vi "Open API Tester.vi"(6 "Run API Tester?":bool, 8 "error in":errorcluster, 10 "Library":refnum<class "Library.lvclass">, 11 "Project":refnum<class "Project.lvclass">) -> (0 "error out":errorcluster)   [LabVIEW 2020, in "Panther Dashboard.lvlib"]
doc: "This VI checks the Main.vi State of the selected DQMH Module"
uses:
  Panther Dashboard.lvlib
  Class/Project/Project.lvclass
  Class/Library/Library.lvclass
  Class/Project/Project.lvclass/Project.ctl
  Class/Library/Library.lvclass/Library.ctl
  Class/Project/Read Main App Inst Ref.vi
  Class/Project/Read Target Name.vi
  Class/Library/Read Library Ref.vi
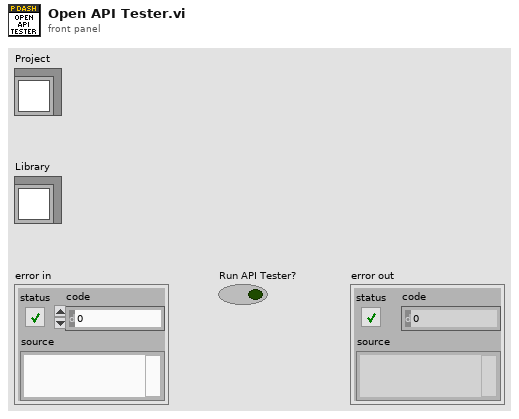
[diagram p1: front panel]
types:
  T1 = enum32{"Bad", "Idle", "Run top level", "Running"}
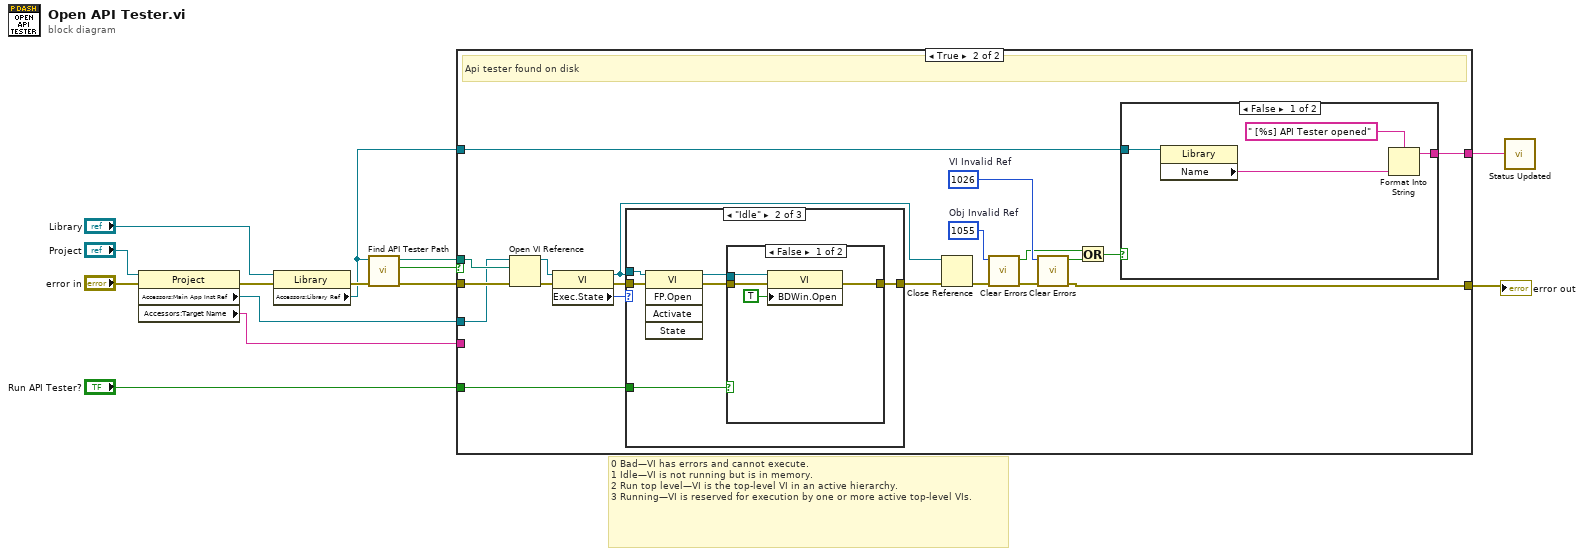
[diagram p0: block diagram]
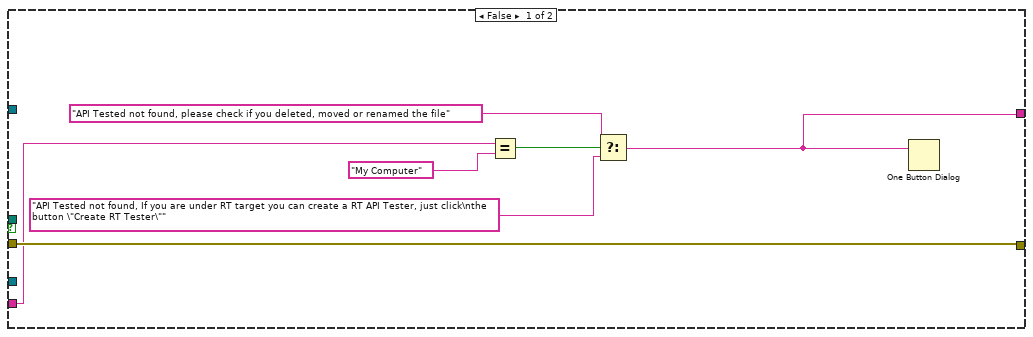
[diagram p2: hidden frame]
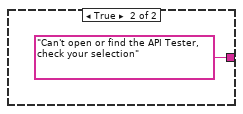
[diagram p3: hidden frame]
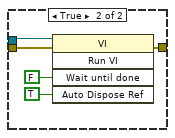
[diagram p5: hidden frame]
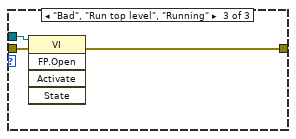
[diagram p6: hidden frame]
diagram:
  # "0\tBad—VI has errors and cannot execute.\n1\tIdle—VI is not running but is in memory.\n2\tRun top level—VI is the top-level VI in an active hierarchy.\n3\tRunning—VI is reserved for execution by one or more active top-level VIs."
  n1 = property class="Project"(reference="Project", error in="error in") -> (error out=w10:errorcluster, "Accessors:Main App Inst Ref"=w3:refnum<vi>, "Accessors:Target Name"=w2:string)  [unwired: 1 out]
  n2 = property class="Library"(reference="Library", error in=w10) -> (error out=w11:errorcluster, "Accessors:Library Ref"=w5:refnum<vi>)  [unwired: 1 out]
  n3 = call "Find API Tester Path.vi"("error in"=w11, "DQMH Library Ref"=w5) -> ("error out"=w13:errorcluster, "Api tester found?"=w8:bool, "API Tester Path"=w9:path)  [unwired: 7 in]
  n4 = case shown="True" w8 {
    tunnel: w13 -> [w21 w40]
    tunnel: w9 -> [_ w34]
    tunnel: w5 -> [_ w25]
    tunnel: w3 -> [_ w24]
    tunnel: [w21 w35] -> w12
    tunnel: [w16 w23] -> w7
    tunnel: w2 -> [w15 _]
    tunnel: "Run API Tester?" -> [_ w22]
    frame False {
      n5 = Equal?(x=w15, y="My Computer") -> (x = y?=w19:bool)
      n6 = Select(t="API Tested not found, please check if you deleted, moved or renamed the file", s=w19, f="API Tested not found, If you are under RT target you can create a RT API Tester, just click\nthe button \"Create RT Tester\"") -> (s? t:f=w16:string)
      n7 = One Button Dialog(message=w16) -> ()  [unwired: 1 in, 1 out]
    }
    frame True {
      w30 = 1055  # Obj Invalid Ref
      w29 = 1026  # VI Invalid Ref
      # "Api tester found on disk"
      n8 = Open VI Reference(application reference (local)=w24, vi path=w34, error in (no error)=w40) -> (vi reference=w33:refnum<vi>, error out=w41:errorcluster)  [unwired: 3 in]
      n9 = property class="VI"(reference=w33, error in=w41) -> (reference out=w31:refnum<vi>, error out=w39:errorcluster, "Exec.State"=w32:T1)
      n10 = case shown="\"Idle\"" w32 {
        tunnel: w31 -> [_ w49 w63]
        tunnel: w39 -> [w47 w52 w64]
        tunnel: [w47 w51 w65] -> w38
        tunnel: w22 -> [_ w48 _]
        frame Default {
        }
        frame "Idle" {
          n11 = invoke class="VI" method="FP.Open"(reference=w49, error in=w52) -> (reference out=w50:refnum<vi>, error out=w53:errorcluster)  [unwired: 3 in, 3 out]
          n12 = case shown="False" w48 {
            tunnel: w53 -> [w57 w62]
            tunnel: [w56 w61] -> w51
            tunnel: w50 -> [w55 w60]
            frame False {
              n13 = property class="VI"(reference=w55, error in=w57, "BDWin.Open"=TRUE ("Block Diagram Window:Open")) -> (error out=w56:errorcluster)  [unwired: 1 out]
            }
            frame True {
              n14 = invoke class="VI" method="Run VI"(reference=w60, error in=w62, "Wait until done"=FALSE ("Wait Until Done"), "Auto Dispose Ref"=TRUE ("Auto Dispose Reference")) -> (error out=w61:errorcluster)  [unwired: 1 in, 4 out]
            }
          }
        }
        frame "Bad", "Run top level", "Running" {
          n15 = invoke class="VI" method="FP.Open"(reference=w63, error in=w64) -> (error out=w65:errorcluster)  [unwired: 3 in, 4 out]
        }
      }
      n16 = Close Reference(reference=w31, error in (no error)=w38) -> (error out=w37:errorcluster)
      n17 = call <vilib>:"Clear Errors.vi"("error in (no error)"=w37, "specific error code to clear (0: all)"=w30) -> ("error out"=w36:errorcluster, "specific error cleared?"=w28:bool)  [unwired: 4 in]
      n18 = call <vilib>:"Clear Errors.vi"("error in (no error)"=w36, "specific error code to clear (0: all)"=w29) -> ("error out"=w35:errorcluster, "specific error cleared?"=w27:bool)  [unwired: 4 in]
      n19 = Or(x=w28, y=w27) -> (x .or. y?=w26:bool)
      n20 = case shown="False" w26 {
        tunnel: w25 -> [w43 _]
        tunnel: [w42 "Can't open or find the API Tester, check your selection"] -> w23
        frame False {
          n21 = property on="Property Node" class="Library"(reference=w43) -> ("Name"=w44:string)  [unwired: 1 in, 2 out]
          n22 = Format Into String(format string=" [%s] API Tester opened" ("Status"), w44) -> (resulting string=w42:string)  [unwired: 2 in, 1 out]
        }
        frame True {
        }
      }
    }
  }
  "error out" <- w12
  n23 = call "Status Updated.vi"("Status"=w7) -> ()  [unwired: 10 in, 1 out]
